vi "AcquireHardware.vi"(8 "error in (no error)":errorcluster, 10 "Axis 1":string, 11 "XPS-RLD in":refnum<class "XPS-RLD.lvclass">) -> (0 "error out":errorcluster, 3 "Current position (units)":dbl)   [LabVIEW 2020, in "XPS-RLD.lvclass"]
uses:
  XPS-RLD.lvclass
  XPS-RLD.lvclass/XPS-RLD.ctl
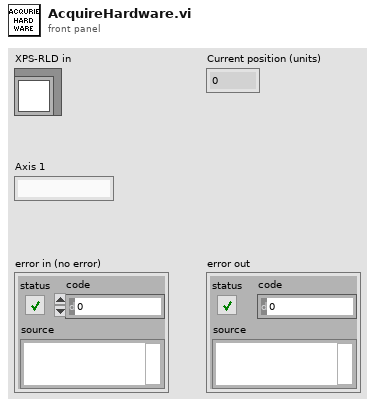
[diagram p1: front panel]
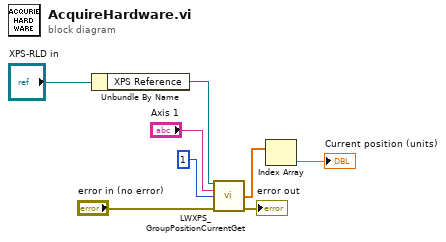
[diagram p0: block diagram]
diagram:
  n1 = Unbundle By Name("XPS-RLD in") -> ("XPS Reference"=w1:refnum<k24>)
  n2 = call "LWXPS_GroupPositionCurrentGet.vi"("XPS Reference IN"=w1, "Group Name"="Axis 1", "Number of positioners"=1, "LabVIEW error IN"="error in (no error)") -> ("Current Encoder Position"=w5:dbl[], "LabVIEW error OUT"=→"error out":errorcluster)  [unwired: 7 in, 3 out]
  n3 = Index Array(array=w5) -> (element=→"Current position (units)":dbl)  [unwired: 1 in]
